vi "Heart Rate Monitor.vi"() -> ()   [LabVIEW 2020]
doc: "The Heart Rate Monitor application that is composed of three major sections: <b>Data Acquisition</b>, <b>Data Processing</b>, and <b>Data Presentation</b>."
uses:
  Controls/Detect Threshold Control.ctl
panel:
  out "Bradicardia":bool
  out "Taquicardia":bool
  out "Waveform Chart":dynamicdata(graph)
  out "Data":dynamicdata(graph) caption="Monitor de batimento cardíaco"
  out "BPM":string="Calibrating..."
  in  "Simular batimento cardíaco?":bool caption="Simulate?"
  in  "Stop":bool
  out "Pulso":bool
  # "MUDAR Y-SCALE CONSOANTE ESTAMOS\nNO SIMULADO OU NÃO"
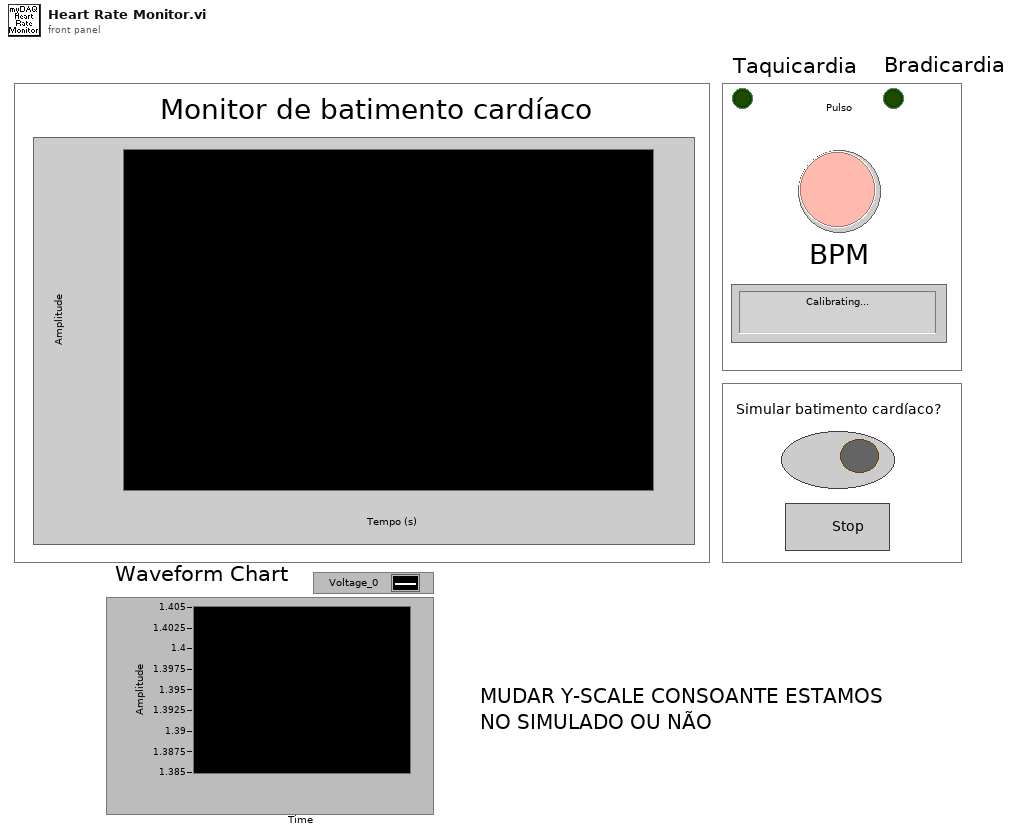
[diagram p1: front panel]
types:
  T1 = typedef "Detect Threshold Control.ctl" = enum16{"Get Threshold", "Pulse Found", "Pulse Not Found"}
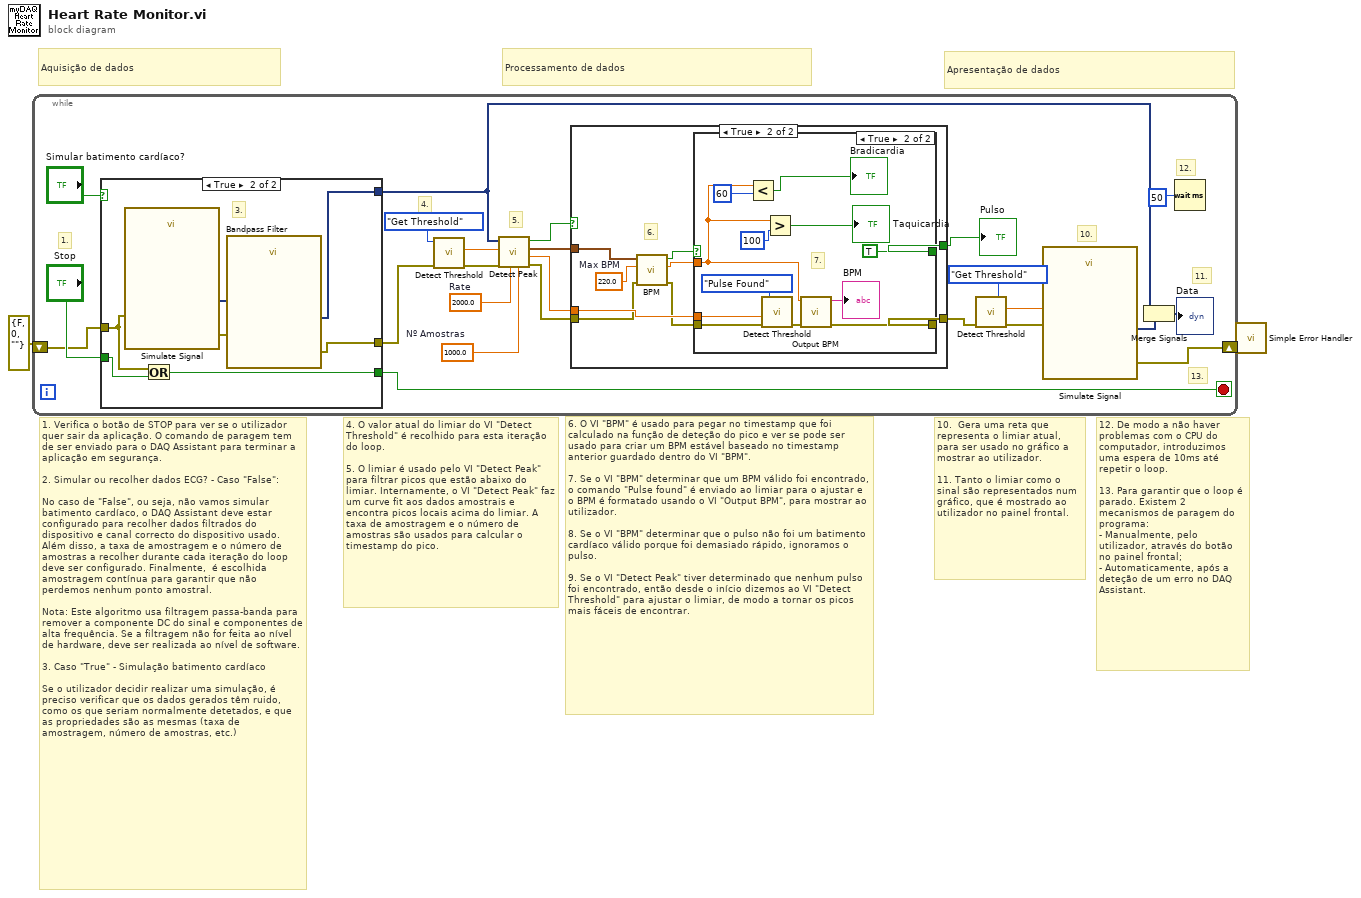
[diagram p0: block diagram]
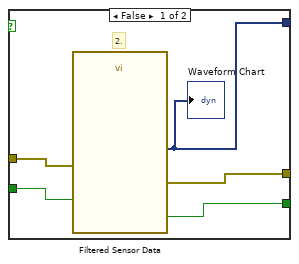
[diagram p2: hidden frame]
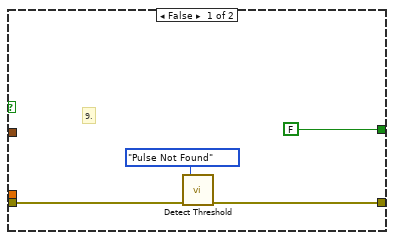
[diagram p3: hidden frame]
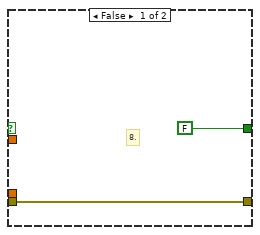
[diagram p4: hidden frame]
diagram:
  # "Apresentação de dados"
  # "Processamento de dados"
  # "Aquisição de dados"
  # "12. De modo a não haver problemas com o CPU do computador, introduzimos uma espera de 10ms até repetir o loop.\n\n13. Para garantir que o loop é parado. Existem 2 mecanismos de paragem do programa:\n- Manualmente, pelo utilizador, através do botão no painel frontal;\n- Automaticamente, após a deteção de um erro no DAQ Assistant."
  # "10.  Gera uma reta que representa o limiar atual, para ser usado no gráfico a mostrar ao utilizador.\n\n11. Tanto o limiar como o sinal são representados num gráfico, que é mostrado ao utilizador no painel frontal."
  # "6. O VI \"BPM\" é usado para pegar no timestamp que foi calculado na função de deteção do pico e ver se pode ser usado para criar um BPM estável baseado no timestamp anterior guardado dentro do VI \"BPM\".\n\n7. Se o VI \"BPM\" determinar que um BPM válido foi encontrado, o comando \"Pulse found\" é enviado ao limiar para o ajustar e o BPM é formatado usando o VI \"Output BPM\", para mostrar ao utilizador.\n\n8. Se o VI \"BPM\" determinar que o pulso não foi um batimento cardíaco válido porque foi demasiado rápido, ignoramos o pulso.\n\n9. Se o VI \"Detect Peak\" tiver determinado que nenhum pulso foi encontrado, então desde o início dizemos ao VI \"Detect Threshold\" para ajustar o limiar, de modo a tornar os picos mais fáceis de encontrar."
  # "4. O valor atual do limiar do VI \"Detect Threshold\" é recolhido para esta iteração do loop.\n\n5. O limiar é usado pelo VI \"Detect Peak\" para filtrar picos que estão abaixo do limiar. Internamente, o VI \"Detect Peak\" faz um curve fit aos dados amostrais e encontra picos locais acima do limiar. A taxa de amostragem e o número de amostras são usados para calcular o timestamp do pico."
  # "1. Verifica o botão de STOP para ver se o utilizador quer sair da aplicação. O comando de paragem tem de ser enviado para o DAQ Assistant para terminar a aplicação em segurança.\n\n2. Simular ou recolher dados ECG? - Caso \"False\":\n\nNo caso de \"False\", ou seja, não vamos simular batimento cardíaco, o DAQ Assistant deve estar configurado para recolher dados filtrados do dispositivo e canal correcto do dispositivo usado. Além disso, a taxa de amostragem e o número de amostras a recolher durante cada iteração do loop deve ser configurado. Finalmente,  é escolhida amostragem contínua para garantir que não perdemos nenhum ponto amostral. \n\nNota: Este algoritmo usa filtragem passa-banda para remover a componente DC do sinal e componentes de alta frequência. Se a filtragem não for feita ao nível de hardware, deve ser realizada ao nível de software.\n\n3. Caso \"True\" - Simulação batimento cardíaco\n\nSe o utilizador decidir realizar uma simulação, é preciso verificar que os dados gerados têm ruido, como os que seriam normalmente detetados, e que as propriedades são as mesmas (taxa de amostragem, número de amostras, etc.)"
  n1 = while {
    shift-right: [w5] -> w2
    shift-left: errorcluster {"status"=FALSE, "code"=0, "source"=""} ("error out") -> [w13]
    stop <- w4 stop-if-true
    w14 = 1000.0  # Nº Amostras
    w15 = 2000.0  # Rate
    # "5."
    # "13."
    # "12."
    # "11."
    # "10."
    # "4."
    # "1."
    n2 = case shown="True" "Simular batimento cardíaco?" {
      tunnel: [w31 w32] -> w4
      tunnel: "Stop" -> [w30 w34]
      tunnel: [w27 w38] -> w3
      tunnel: [w28 w35] -> w9
      tunnel: w13 -> [w29 w33]
      frame False {
        # "2."
        n3 = call "Filtered Sensor Data"("error in"=w29, "stop (F)"=w30) -> ("data"=w27:dynamicdata, "stopped"=w31:bool, "error out"=w28:errorcluster)  [unwired: 14 in, 1 out]
        "Waveform Chart" <- w27
      }
      frame True {
        # "3."
        n4 = call "Simulate Signal"("error in (no error)"=w33) -> ("Simulated Sensor"=w37:dynamicdata, "error out"=w36:errorcluster)  [unwired: 13 in]
        n5 = Or(x=w33, y=w34) -> (x .or. y?=w32:bool)
        n6 = call "Bandpass Filter"("error in (no error)"=w36, "Signal"=w37) -> ("error out"=w35:errorcluster, "Filtered Signal"=w38:dynamicdata)  [unwired: 8 in]
      }
    }
    n7 = call "Detect Threshold.vi"("error in (no error)"=w9, "Action"=Detect_Threshold_Control."Get Threshold") -> ("error out"=w17:errorcluster, "Threshold"=w18:dbl)  [unwired: 4 in]
    n8 = call "Detect Peak.vi"("Num Samples"=w14, "Rate"=w15, "error in (no error)"=w17, "Threshold"=w18, "Filtered Signal"=w3) -> ("error out"=w16:errorcluster, "Peak Amplitude"=w22:dbl, "Peak Time Stamp"=w23:timestamp, "Peak Found?"=w12:bool)  [unwired: 3 in]
    n9 = case shown="True" w12 {
      tunnel: w23 -> [_ w51]
      tunnel: w22 -> [_ w49]
      tunnel: w16 -> [w41 w43]
      tunnel: [w40 w46] -> w8
      tunnel: [FALSE w44] -> w10
      frame False {
        # "9."
        n10 = call "Detect Threshold.vi"("error in (no error)"=w41, "Action"=Detect_Threshold_Control."Pulse Not Found") -> ("error out"=w40:errorcluster)  [unwired: 4 in, 1 out]
      }
      frame True {
        w50 = 220.0  # Max BPM
        # "6."
        n11 = call "BPM.vi"("error in (no error)"=w43, "Max BPM Threshold"=w50, "Time Stamp"=w51) -> ("error out"=w45:errorcluster, "BPM"=w47:dbl, "Below MAX BPM Threshold?"=w48:bool)  [unwired: 2 in]
        n12 = case shown="True" w48 {
          tunnel: w49 -> [_ w65]
          tunnel: w47 -> [_ w58]
          tunnel: [w53 w62] -> w46
          tunnel: w45 -> [w53 w61]
          tunnel: [FALSE TRUE] -> w44
          frame False {
            # "8."
          }
          frame True {
            # "7."
            n13 = Less?(x=w58, y=60) -> (x < y?=→"Bradicardia":bool)
            n14 = call "Detect Threshold.vi"("error in (no error)"=w61, "Amplitude"=w65, "Action"=Detect_Threshold_Control."Pulse Found") -> ("error out"=w63:errorcluster)  [unwired: 3 in, 1 out]
            n15 = Greater?(x=w58, y=100) -> (0:→"Taquicardia":bool)
            n16 = call "Output BPM.vi"("error in (no error)"=w63, "BPM (input)"=w58) -> ("error out"=w62:errorcluster, "BPM (output)"=→"BPM":string)  [unwired: 4 in]
          }
        }
      }
    }
    "Pulso" <- w10
    n17 = call "Detect Threshold.vi"("error in (no error)"=w8, "Action"=Detect_Threshold_Control."Get Threshold") -> ("error out"=w7:errorcluster, "Threshold"=w19:dbl)  [unwired: 4 in]
    n18 = call "Simulate Signal"("Offset"=w19, "error in (no error)"=w7) -> ("Limiar do pico"=w11:dynamicdata, "error out"=w5:errorcluster)  [unwired: 12 in]
    n19 = Merge Signals(w3, w11) -> (→"Data":dynamicdata)
    n20 = Wait (ms)(milliseconds to wait=u32 50) -> ()  [unwired: 1 out]
  }
  n21 = call <vilib>:"Simple Error Handler.vi"("error in (no error)"=w2) -> ()  [unwired: 4 in, 5 out]
